vi "Set Axis Speed.vi"(8 "error in (no error)":errorcluster, 9 "Speed (mm/s)":dbl=1.0, 10 "Axis":T1, 11 "VISA resource name":refnum<visa-resource-name>) -> (0 "error out":errorcluster, 3 "VISA out":refnum<visa-resource-name>)   [LabVIEW 2017, in "Drivers.lvlib" / "ASI TG-1000.lvlib"]
uses:
  ASI TG-1000.lvlib
  Utility/Axis Name.ctl
  Utility/Serial Response Syntax.ctl
panel:
  out "Command":string
  out "Command Accepted?":bool
  out "Response":string
  # "NB: this VI opens and closes the comm port"
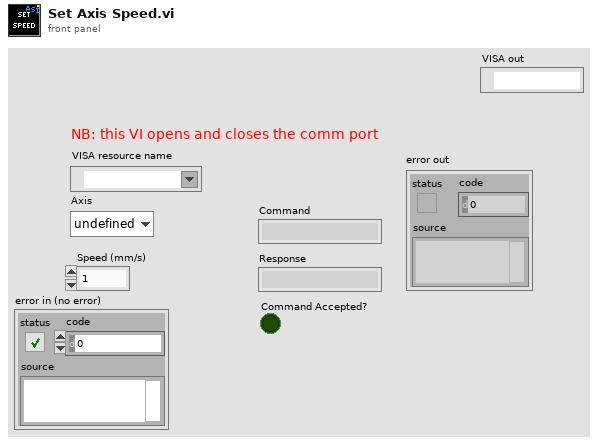
[diagram p1: front panel]
types:
  T1 = typedef "Drivers.lvlib/ASI TG-1000.lvlib/Axis Name.ctl" = enum8{"undefined", "A", "B", "C", "D", "E", "F", "G", "H", "I", "J", "K", "L", "M", "N", "O", "P", "Q", "R", "S", "T", "U", "V", "W", "X", "Y", "Z"}
  T2 = typedef "Drivers.lvlib/ASI TG-1000.lvlib/Serial Response Syntax.ctl" = enum16{":A then single line", "Single line, no :A", ":A or : then single line", ":A then single number", ":A or : then single number", ":A then <axis>= single number"}
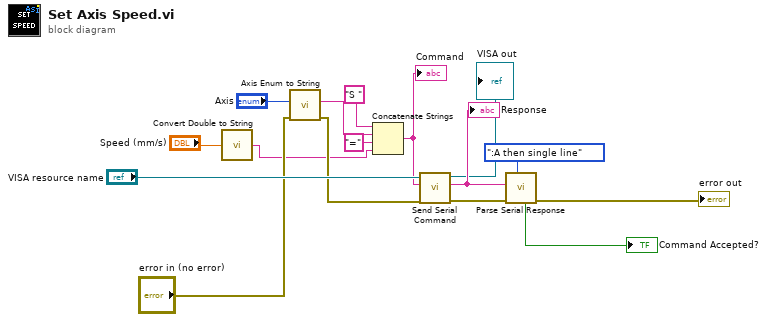
[diagram p0: block diagram]
diagram:
  n1 = call "Convert Double to String.vi"("Value"="Speed (mm/s)") -> ("String"=w3:string)
  n2 = call "Axis Enum to String.vi"("error in (no error)"="error in (no error)", "Axis Enum In"="Axis") -> ("error out"=w12:errorcluster, "Axis String Out"=w11:string)  [unwired: 8 in]
  n3 = Concatenate Strings("S " ("Command"), w11, "=" ("string"), w3) -> (w9:string)
  "Command" <- w9
  n4 = call "Send Serial Command.vi"("error in (no error)"=w12, "Command"=w9, "VISA in"="VISA resource name") -> ("error out"=w7:errorcluster, "Response"=w5:string, "VISA out"=→"VISA out":refnum<visa-resource-name>)  [unwired: 6 in]
  "Response" <- w5
  n5 = call "Parse Serial Response.vi"("Response Syntax"=Serial_Response_Syntax.":A then single line", "error in (no error)"=w7, "Raw Response"=w5) -> ("error out"=→"error out":errorcluster, "As expected?"=→"Command Accepted?":bool)  [unwired: 5 in, 2 out]
